vi "Refresh Continuous Controls.vi"(8 "error in":errorcluster caption="错误输入（无错误）", 10 "Cmd":T1, 11 "Ctrls":T2) -> (0 "error out":errorcluster caption="错误输出")   [LabVIEW 2016]
uses:
  Ctrls/Continuous Operations.ctl
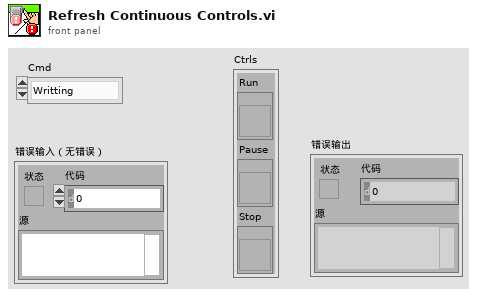
[diagram p1: front panel]
types:
  T1 = typedef "Continuous Operations.ctl" = enum16{"Writting", "Pause", "Stop"}
  T2 = cluster{"Run":refnum<vi>, "Pause":refnum<vi>, "Stop":refnum<vi>}
  T3 = enum8{"Enabled", "Disabled", "Disabled and Grayed Out"}
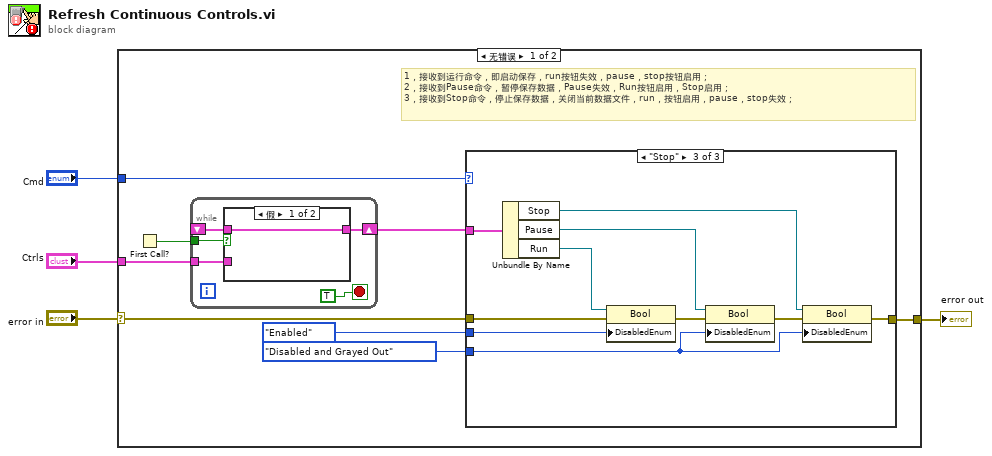
[diagram p0: block diagram]
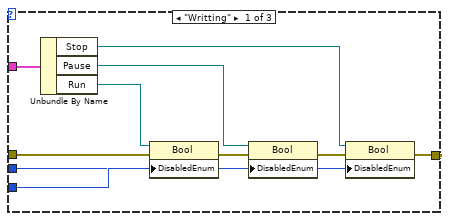
[diagram p3: hidden frame]
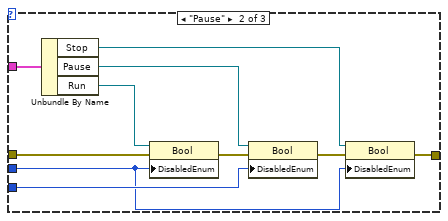
[diagram p4: hidden frame]
diagram:
  n1 = case shown="无错误" "error in" {
    selector: "error in" -> [w8 w50]
    tunnel: [w10 w50] -> w3
    tunnel: "Ctrls" -> [w6 _]
    tunnel: "Cmd" -> [w9 _]
    frame No Error {
      # "1，接收到运行命令，即启动保存，run按钮失效，pause，stop按钮启用；\n2，接收到Pause命令，暂停保存数据，Pause失效，Run按钮启用，Stop启用；\n3，接收到Stop命令，停止保存数据，关闭当前数据文件，run，按钮启用，pause，stop失效；"
      n2 = First Call?() -> (First Call?: T/F=w7:bool)
      n3 = while {
        shift-right: [w14] -> w5
        shift-left: _ -> [w15]
        tunnel: w7 -> [w16]
        tunnel: w6 -> [w13]
        stop <- TRUE stop-if-true
        n4 = case shown="假" w16 {
          tunnel: w15 -> [w18 _]
          tunnel: [w18 w19] -> w14
          tunnel: w13 -> [_ w19]
          frame False {
          }
          frame True {
          }
        }
      }
      n5 = case shown="\"Stop\"" w9 {
        tunnel: w8 -> [w28 w38 w48]
        tunnel: w5 -> [w29 w39 w49]
        tunnel: T3."Enabled" ("Disabled") -> [w21 w30 w41]
        tunnel: T3."Disabled and Grayed Out" ("Disabled") -> [w22 w31 w40]
        tunnel: [w20 w32 w42] -> w10
        frame "Writting" {
          n6 = Unbundle By Name(w29) -> ("Stop"=w23:refnum<vi>, "Pause"=w25:refnum<vi>, "Run"=w27:refnum<vi>)
          n7 = property class="Bool"(reference=w27, error in=w28, "DisabledEnum"=w22) -> (error out=w26:errorcluster)  [unwired: 1 out]
          n8 = property class="Bool"(reference=w25, error in=w26, "DisabledEnum"=w21) -> (error out=w24:errorcluster)  [unwired: 1 out]
          n9 = property class="Bool"(reference=w23, error in=w24, "DisabledEnum"=w21) -> (error out=w20:errorcluster)  [unwired: 1 out]
        }
        frame "Pause" {
          n10 = Unbundle By Name(w39) -> ("Stop"=w33:refnum<vi>, "Pause"=w35:refnum<vi>, "Run"=w37:refnum<vi>)
          n11 = property class="Bool"(reference=w37, error in=w38, "DisabledEnum"=w30) -> (error out=w36:errorcluster)  [unwired: 1 out]
          n12 = property class="Bool"(reference=w35, error in=w36, "DisabledEnum"=w31) -> (error out=w34:errorcluster)  [unwired: 1 out]
          n13 = property class="Bool"(reference=w33, error in=w34, "DisabledEnum"=w30) -> (error out=w32:errorcluster)  [unwired: 1 out]
        }
        frame "Stop" {
          n14 = Unbundle By Name(w49) -> ("Stop"=w43:refnum<vi>, "Pause"=w45:refnum<vi>, "Run"=w47:refnum<vi>)
          n15 = property class="Bool"(reference=w47, error in=w48, "DisabledEnum"=w41) -> (error out=w46:errorcluster)  [unwired: 1 out]
          n16 = property class="Bool"(reference=w45, error in=w46, "DisabledEnum"=w40) -> (error out=w44:errorcluster)  [unwired: 1 out]
          n17 = property class="Bool"(reference=w43, error in=w44, "DisabledEnum"=w40) -> (error out=w42:errorcluster)  [unwired: 1 out]
        }
      }
    }
    frame Error {
    }
  }
  "error out" <- w3
